vi "testest.vi"() -> ()   [LabVIEW 2019]
uses:
  <vilib>/WPC Systems Ltd/GECO Driver/Lib/GECOMotion/GECOMotion/_typedefine/Axis Select.ctl
  <vilib>/WPC Systems Ltd/GECO Driver/Lib/GECOBase/GECO_Driver Class/Motion/_typedefine/GECO_Stepper Output Configuration.ctl
  <vilib>/WPC Systems Ltd/GECO Driver/Lib/GECOBase/GECO_Driver Class/Motion/_typedefine/GECO_Motion Operation Mode.ctl
  <vilib>/WPC Systems Ltd/GECO Driver/Lib/GECOBase/GECO_Driver Class/GECO_SlotName.ctl
  <vilib>/WPC Systems Ltd/GECO Driver/Lib/GECOBase/GECO_Driver Class/Motion/_typedefine/GECO_ActiveHighLow.ctl
  <vilib>/WPC Systems Ltd/GECO Driver/GECODriver/GECO_Initialize_PC/Initialize VIs/Initialize_GECOUno_4HX.vi
  <vilib>/WPC Systems Ltd/GECO Driver/Lib/GECOBase/GECO_Driver Class/GECO_Driver.lvclass
  <vilib>/WPC Systems Ltd/GECO Driver/Lib/GECOMotion/GECOMotion/GECO Motion.lvclass
panel:
  in  "resource name":tag
  in  "Reverse Polarity 2":T1=enum."Active Low"
  in  "Forward Polarity 2":T1=enum."Active Low"
  in  "Motion Controller Slot 2":T2
  in  "Motion Operation Mode 2":T3
  in  "Deacceleration (100000) 2":u32=100000
  in  "Acceleration (100000) 2":u32=100000
  in  "Velocity (10000) 2":i32=10000 min=-20000000 max=20000000
  in  "Target Position (0) 2":i32=1000
  in  "Reverse Enable? 2":bool
  in  "Forward Enable? 2":bool=TRUE
  in  "Stepper Output Configuration 2":T4
  in  "Axis Select 2":T5
  out "Move Complete?":bool
  out "Logical Position":i32
  out "Encoder Position":i32
  in  "Shoot":bool
  in  "Reverse Polarity":T1=enum."Active Low"
  in  "Forward Polarity":T1=enum."Active Low"
  in  "Motion Controller Slot":T2
  in  "Motion Operation Mode":T3
  in  "Deacceleration (100000)":u32=100000
  in  "Acceleration (100000)":u32=100000
  in  "Velocity (10000)":i32=10000 min=-20000000 max=20000000
  in  "Target Position (0)":i32=1000
  in  "Reverse Enable?":bool
  in  "Forward Enable?":bool=TRUE
  in  "Stepper Output Configuration":T4
  in  "Axis Select":T5
  out "LED":bool
  out "text":string
  out "MainProgramQueue 2":string
  in  "MainProgramQueue":string
  in  "stop":bool
  in  "Button":bool
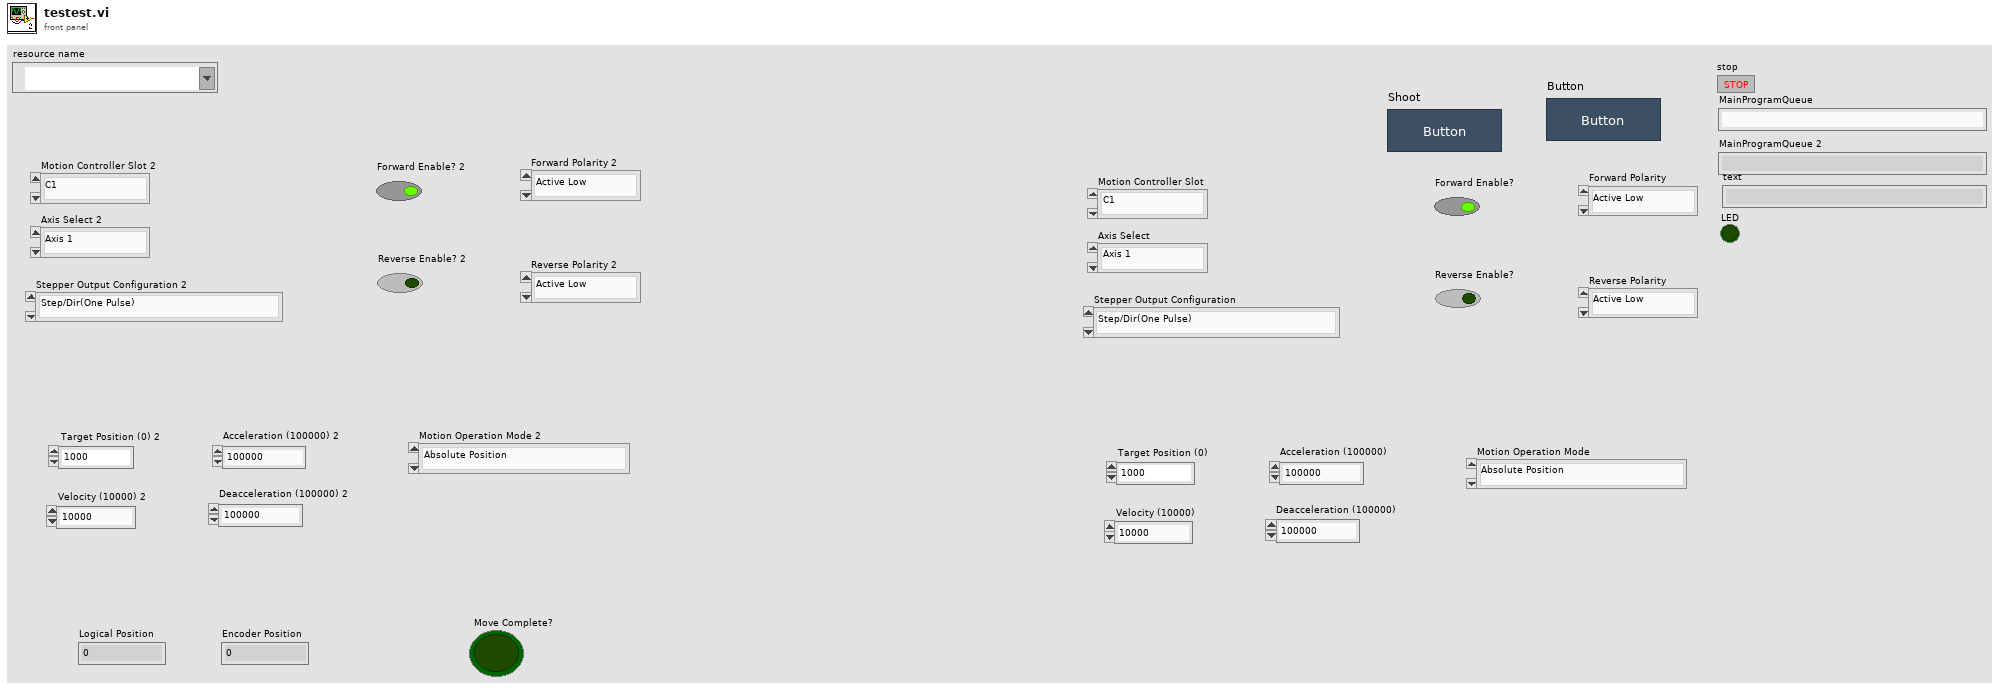
[diagram p1: front panel]
types:
  T1 = typedef "GECO_Driver.lvclass/GECO_ActiveHighLow.ctl" = enum16{"Active High", "Active Low"}
  T2 = typedef "GECO_Driver.lvclass/GECO_SlotName.ctl" = enum16{"C1", "C2", "C3", "C4"}
  T3 = typedef "GECO_Driver.lvclass/GECO_Motion Operation Mode.ctl" = enum16{"Absolute Position", "Relative Position", "Velocity"}
  T4 = typedef "GECO_Driver.lvclass/GECO_Stepper Output Configuration.ctl" = enum16{"Step/Dir(One Pulse)", "CW/CCW(Two Pulse)"}
  T5 = typedef "GECO Motion.lvclass/Axis Select.ctl" = enum16{"Axis 1", "Axis 2", "Axis 3", "Axis 4"}
  T6 = cluster{"Forward Enable":bool, "Forward Polarity":T1}
  T7 = cluster{"Reverse Enable":bool, "Reverse Polarity":T1}
  T8 = cluster{"Motion Operation Mode":T3, "Target Position (0)":i32, "Velocity (10000)":i32, "Acceleration (100000)":u32, "Deacceleration (100000)":u32}
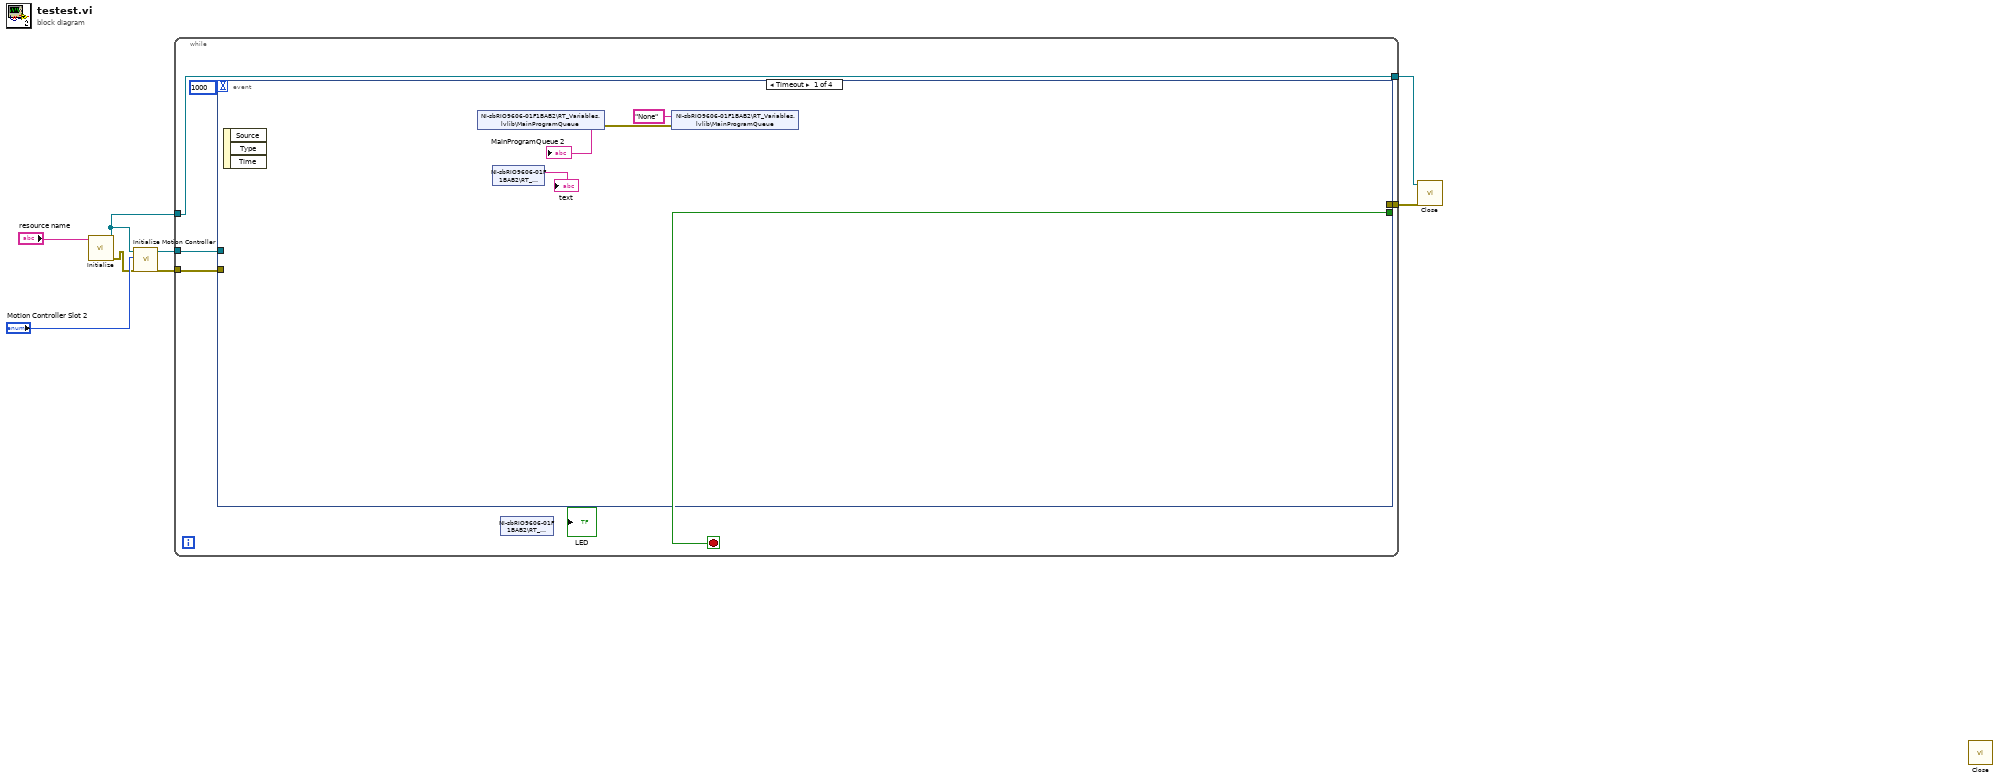
[diagram p0: block diagram]
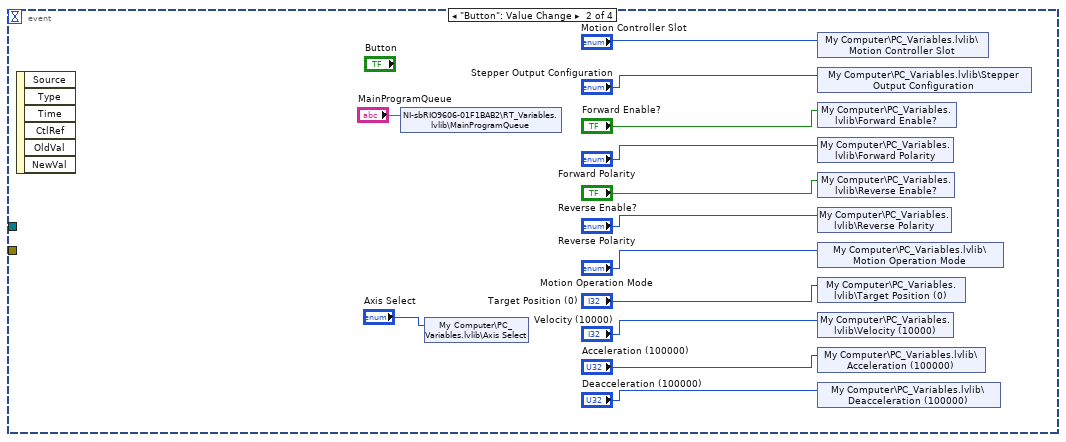
[diagram p2: hidden frame]
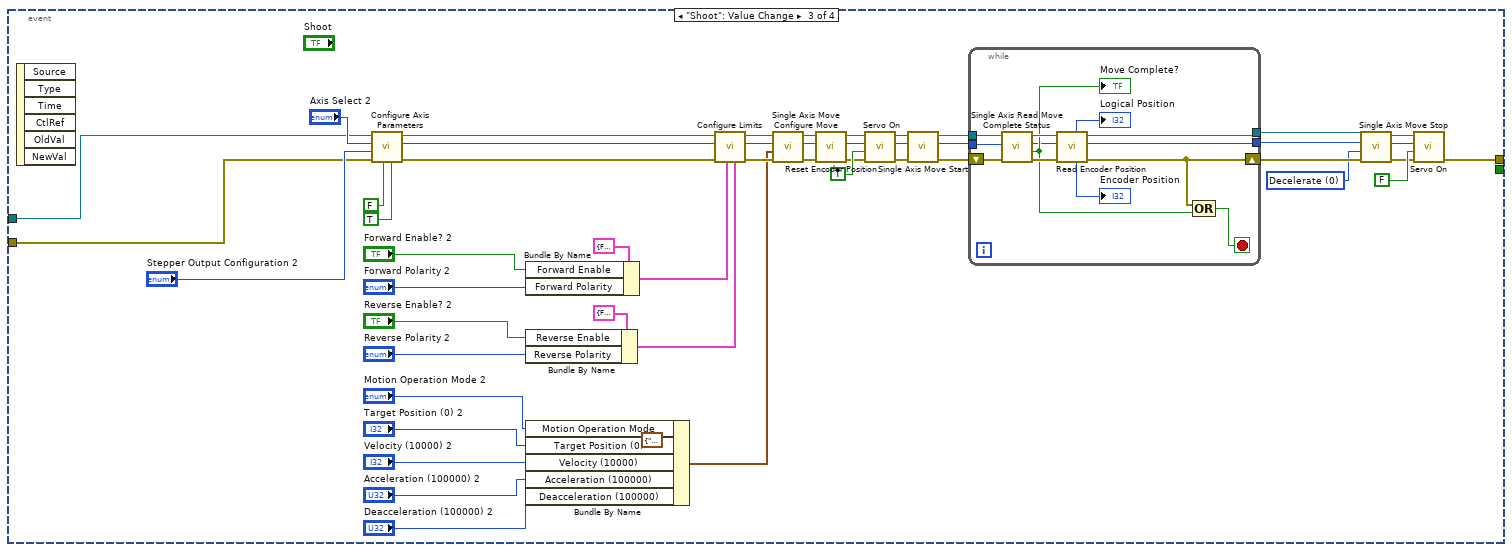
[diagram p3: hidden frame]
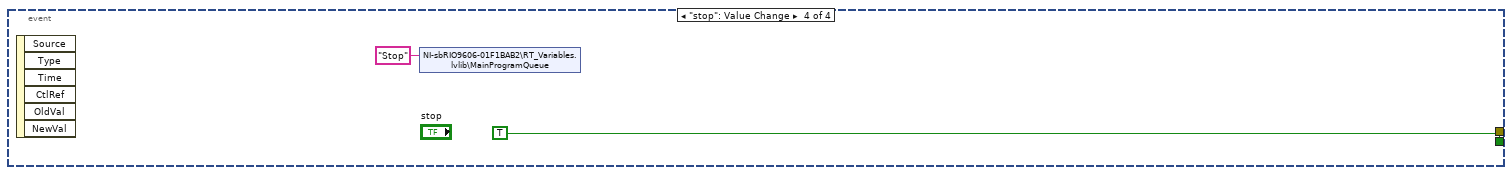
[diagram p4: hidden frame]
diagram:
  n1 = call-poly <vilib>:"Initialize.vi"("resource name"="resource name") -> ("error out"=w2:errorcluster, "GECO_Driver out"=w6:refnum<class "GECO_Driver.lvclass">)  [unwired: 9 in]
  n2 = call <vilib>:"Initialize Motion Controller.vi"("error in (no error)"=w2, "Slot"="Motion Controller Slot 2", "GECO_Driver in"=w6) -> ("error out"=w4:errorcluster, "Motion reference out"=w5:refnum<class "GECO Motion.lvclass">)  [unwired: 7 in]
  n3 = while {
    tunnel: [w12] -> w8
    tunnel: w6 -> [w9]
    tunnel: w4 -> [w11]
    tunnel: w5 -> [w10]
    tunnel: [w9] -> w1
    stop <- w14 stop-if-true
    n4 = event shown="[0] Timeout" {
      selector: _ -> [_ _ _ _]
      dyn-events: _ -> [_ _ _ _]
      timeout: 1000 -> [_ _ _ _]
      tunnel: [_ _ _ TRUE] -> w14
      tunnel: [_ _ w34 _] -> w12
      tunnel: w11 -> [_ _ w33 _]
      tunnel: w10 -> [_ _ w32 _]
      event Timeout {
        n5 = event-data() -> ()  [unwired: 1 in, 3 out]
        n6 = shared-variable "NI-sbRIO9606-01F1BAB2\\RT_Variables.lvlib\\MainProgramQueue"() -> (→"MainProgramQueue 2":string, error out=w16:errorcluster)  [unwired: 1 in]
        n7 = shared-variable "NI-sbRIO9606-01F1BAB2\\RT_Variables.lvlib\\text"() -> (→"text":string)  [unwired: 1 in, 1 out]
        n8 = shared-variable "NI-sbRIO9606-01F1BAB2\\RT_Variables.lvlib\\MainProgramQueue"("None" ("MainProgramQueue"), error in=w16) -> ()  [unwired: 1 out]
      }
      event "Button": Value Change {
        n9 = event-data() -> ()  [unwired: 1 in, 6 out]
        n10 = shared-variable "NI-sbRIO9606-01F1BAB2\\RT_Variables.lvlib\\MainProgramQueue"("MainProgramQueue") -> ()  [unwired: 1 in, 1 out]
        n11 = shared-variable "My Computer\\PC_Variables.lvlib\\Axis Select"("Axis Select") -> ()  [unwired: 1 in, 1 out]
        n12 = shared-variable "My Computer\\PC_Variables.lvlib\\Motion Controller Slot"("Motion Controller Slot") -> ()  [unwired: 1 in, 1 out]
        n13 = shared-variable "My Computer\\PC_Variables.lvlib\\Stepper Output Configuration"("Stepper Output Configuration") -> ()  [unwired: 1 in, 1 out]
        n14 = shared-variable "My Computer\\PC_Variables.lvlib\\Forward Enable?"("Forward Enable?") -> ()  [unwired: 1 in, 1 out]
        n15 = shared-variable "My Computer\\PC_Variables.lvlib\\Forward Polarity"("Forward Polarity") -> ()  [unwired: 1 in, 1 out]
        n16 = shared-variable "My Computer\\PC_Variables.lvlib\\Reverse Enable?"("Reverse Enable?") -> ()  [unwired: 1 in, 1 out]
        n17 = shared-variable "My Computer\\PC_Variables.lvlib\\Reverse Polarity"("Reverse Polarity") -> ()  [unwired: 1 in, 1 out]
        n18 = shared-variable "My Computer\\PC_Variables.lvlib\\Motion Operation Mode"("Motion Operation Mode") -> ()  [unwired: 1 in, 1 out]
        n19 = shared-variable "My Computer\\PC_Variables.lvlib\\Target Position (0)"("Target Position (0)") -> ()  [unwired: 1 in, 1 out]
        n20 = shared-variable "My Computer\\PC_Variables.lvlib\\Velocity (10000)"("Velocity (10000)") -> ()  [unwired: 1 in, 1 out]
        n21 = shared-variable "My Computer\\PC_Variables.lvlib\\Acceleration (100000)"("Acceleration (100000)") -> ()  [unwired: 1 in, 1 out]
        n22 = shared-variable "My Computer\\PC_Variables.lvlib\\Deacceleration (100000)"("Deacceleration (100000)") -> ()  [unwired: 1 in, 1 out]
      }
      event "Shoot": Value Change {
        w73 = u16 0 items=["Decelerate", "Halt"] ("Motion Stop Type")
        n23 = event-data() -> ()  [unwired: 1 in, 6 out]
        n24 = call <vilib>:"Configure Axis Parameters.vi"("Reverse Encoder Direction?"=TRUE ("Encoder Direction"), "Reverse Axis Direction?"=FALSE ("Axis Direction"), "error in (no error)"=w33, "Stepper Output Configuration"="Stepper Output Configuration 2", "Axis Select"="Axis Select 2", "GECO Motion in"=w32) -> ("error out"=w66:errorcluster, "Axis Select out"=w42:T5, "GECO Motion out"=w67:refnum<class "GECO Motion.lvclass">)  [unwired: 3 in]
        n25 = Bundle By Name(cluster=T6 {"Forward Enable"=FALSE, "Forward Polarity"=enum."Active Low"} ("Forward"), "Forward Enable"="Forward Enable? 2", "Forward Polarity"="Forward Polarity 2") -> (w49:T6)
        n26 = Bundle By Name(cluster=T7 {"Reverse Enable"=FALSE, "Reverse Polarity"=enum."Active Low"} ("Reverse"), "Reverse Enable"="Reverse Enable? 2", "Reverse Polarity"="Reverse Polarity 2") -> (w45:T7)
        n27 = Bundle By Name(cluster=T8 {"Motion Operation Mode"=enum."Absolute Position", "Target Position (0)"=0, "Velocity (10000)"=10000, "Acceleration (100000)"=100000, "Deacceleration (100000)"=100000} ("Singel Axis Move Paramters"), "Motion Operation Mode"="Motion Operation Mode 2", "Target Position (0)"="Target Position (0) 2", "Velocity (10000)"="Velocity (10000) 2", "Acceleration (100000)"="Acceleration (100000) 2", "Deacceleration (100000)"="Deacceleration (100000) 2") -> (w60:T8)
        n28 = call <vilib>:"Configure Limits.vi"("Reverse"=w45, "Forward"=w49, "error in (no error)"=w66, "Axis Select"=w42, "GECO Motion in"=w67) -> ("error out"=w64:errorcluster, "Axis Select out"=w41:T5, "GECO Motion out"=w65:refnum<class "GECO Motion.lvclass">)  [unwired: 4 in]
        n29 = call <vilib>:"Single Axis Move Configure Move.vi"("error in (no error)"=w64, "Singel Axis Move Paramters"=w60, "Axis Select"=w41, "GECO Motion in"=w65) -> ("error out"=w62:errorcluster, "Axis Select out"=w40:T5, "GECO Motion out"=w63:refnum<class "GECO Motion.lvclass">)  [unwired: 5 in]
        n30 = call <vilib>:"Reset Encoder Position.vi"("error in (no error)"=w62, "Axis Select"=w40, "GECO Motion in"=w63) -> ("error out"=w68:errorcluster, "Axis Select out"=w39:T5, "GECO Motion out"=w69:refnum<class "GECO Motion.lvclass">)  [unwired: 6 in]
        n31 = call <vilib>:"Servo On.vi"("error in (no error)"=w68, "Servo On"=TRUE, "Axis Select"=w39, "GECO Motion in"=w69) -> ("error out"=w78:errorcluster, "Axis Select out"=w38:T5, "GECO Motion out"=w79:refnum<class "GECO Motion.lvclass">)  [unwired: 5 in]
        n32 = call <vilib>:"Single Axis Move Start.vi"("error in (no error)"=w78, "Axis Select"=w38, "GECO Motion in"=w79) -> ("error out"=w76:errorcluster, "Axis Select out"=w37:T5, "GECO Motion out"=w77:refnum<class "GECO Motion.lvclass">)  [unwired: 6 in]
        n33 = while {
          tunnel: w77 -> [w87]
          tunnel: [w92] -> w75
          shift-right: [w89] -> w74
          shift-left: w76 -> [w88]
          tunnel: w37 -> [w83]
          tunnel: [w81] -> w36
          stop <- w93 stop-if-true
          n34 = call <vilib>:"Single Axis Read Move Complete Status.vi"("error in (no error)"=w88, "Axis Select"=w83, "GECO Motion in"=w87) -> ("error out"=w90:errorcluster, "Move Complete?"=w86:bool, "Axis Select out"=w82:T5, "GECO Motion out"=w91:refnum<class "GECO Motion.lvclass">)  [unwired: 5 in]
          "Move Complete?" <- w86
          n35 = call <vilib>:"Read Encoder Position.vi"("error in (no error)"=w90, "Axis Select"=w82, "GECO Motion in"=w91) -> ("error out"=w89:errorcluster, "Axis Select out"=w81:T5, "GECO Motion out"=w92:refnum<class "GECO Motion.lvclass">, "Encoder Position"=→"Encoder Position":i32, "Logical Position"=→"Logical Position":i32)  [unwired: 4 in]
          n36 = Compound Arithmetic op=OR(w89, w86) -> (w93:bool)
        }
        n37 = call <vilib>:"Single Axis Move Stop.vi"("error in (no error)"=w74, "Motion Stop Type"=w73, "Axis Select"=w36, "GECO Motion in"=w75) -> ("error out"=w70:errorcluster, "Axis Select out"=w35:T5, "GECO Motion out"=w71:refnum<class "GECO Motion.lvclass">)  [unwired: 5 in]
        n38 = call <vilib>:"Servo On.vi"("error in (no error)"=w70, "Servo On"=FALSE, "Axis Select"=w35, "GECO Motion in"=w71) -> ("error out"=w34:errorcluster)  [unwired: 5 in, 2 out]
      }
      event "stop": Value Change {
        n39 = event-data() -> ()  [unwired: 1 in, 6 out]
        n40 = shared-variable "NI-sbRIO9606-01F1BAB2\\RT_Variables.lvlib\\MainProgramQueue"("Stop" ("MainProgramQueue")) -> ()  [unwired: 1 in, 1 out]
      }
    }
    n41 = shared-variable "NI-sbRIO9606-01F1BAB2\\RT_Variables.lvlib\\LED"() -> ()  [unwired: 1 in, 2 out]
  }
  n42 = call <vilib>:"Close.vi"("error in (no error)"=w8, "GECO_Driver in"=w1) -> ()  [unwired: 9 in, 1 out]
  n43 = call <vilib>:"Close.vi"() -> ()  [unwired: 11 in, 1 out]
